vi "Injection.Capture.vi"(7 "FIFOs":T2={"Data Buffer FIFO"="Intermediate Voltage 0", "Capture Complete Trigger FIFO"="Event Capture 0"}, 8 "Current (PreScaled)":fxp<+/-,32,8>, 9 "Voltage (PreScaled)":fxp<+/-,32,8>, 10 "Settings.Index<#>.<Group>.<UserName>":T1, 11 "Settings.Global.<Group>":T3={"Enable?"=FALSE, "Initial Voltage Threshold"=12.0, "Event Dwell Limit"=2000, "Voltage Gain"=1.0, "Current Gain"=1.0, "Filter Samples"=5, "Pretrigger Samples"=5, "Active Edge"=TRUE}) -> (0 "Current (Scaled)":fxp<+/-,32,8>, 1 "Voltage (Scaled)":fxp<+/-,32,8>, 3 "Intermediate FIFO Timeout?":bool)   [LabVIEW 2019]
uses:
  Types/Injection.Global.Settings.ctl
  Types/Injection.Core.Internal.Settings.ctl
  Types/Injection.Core.Settings.ctl
  Types/Injection.Core.State.ctl
  <vilib>/rvi/Emulation/niFpgaSctlEmulationGetInTimedLoop.vi
  <vilib>/Utility/error.llb/Clear Errors.vi
  <vilib>/rvi/DataTransferAndStorage/Container/Common/niFpgaContainerExecOnDevCompGetState.vi
  <vilib>/rvi/Emulation/niFpgaEmulationIsFPGAContextNoSignature.vi
  <vilib>/rvi/errors/niFpgaSetErrorForExecOnDevCompSimple.vi
  <vilib>/rvi/eio/common/nirviEmuReportErrorAndStop.vi
  <vilib>/rvi/DataTransferAndStorage/Container/Common/niFpgaContainerGetUniqueNameForEmu.vi
  <vilib>/rvi/FIFO/Fifo_Resource/nirvififoEmulationSetSize.vi
  <vilib>/rvi/FIFO/Fifo_Resource/nirviFifoEmulationQueueMgr.vi
  <instcachedir>/0/nirviFifoEmulationQueueMgr_E5CAEC123FF24DC58D834DCA3CDAA9B5.lvgen/nirviFifoEmulationQueueMgr_E5CAEC123FF24DC58D834DCA3CDAA9B5_002.vi
  <vilib>/rvi/FIFO/Fifo_Resource/nirvififoEmulationDetermineInputValidOut.vi
  <vilib>/rvi/FIFO/Fifo_Resource/nirvififoEmulationCreateLock.vi
  <vilib>/rvi/Emulation/niFpgaProcessEmulError.vi
  <vilib>/rvi/FIFO/Fifo_Resource/nirvififoEmulationObtainLock.vi
  <vilib>/rvi/FIFO/Fifo_Resource/nirvififoEmulationReleaseLock.vi
  <vilib>/rvi/occurrence/nirviWaitOnOccurrenceBase.vi
  <vilib>/rvi/errors/nirviReportUnexpectedCaseInternalError.vi
  <vilib>/rvi/errors/nirviReportUnexpectedCaseInternalError (U32).vi
  <vilib>/rvi/interface/RandomDataEmulation/niFpgaRandomDataHandleErrors.vi
  <instcachedir>/0/nirviFifoEmulationQueueMgr_E5CAEC123FF24DC58D834DCA3CDAA9B5.lvgen/nirviFifoEmulationQueueMgr_E5CAEC123FF24DC58D834DCA3CDAA9B5_001.vi
  <vilib>/rvi/FXPMathLib/FxpMul/XNode/nifxpmath_Multiplier.xnode
  <vilib>/rvi/FXPMathLib/FxpAdd/XNode/nifxpmath_Add.xnode
  <vilib>/rvi/DataTransferAndStorage/Container/XNode/niFpgaContainer.xnode
  <vilib>/rvi/FIFO/Fifo_Resource/niFpgaFifoEmulationRefIn.vi
  <vilib>/rvi/FXPMathLib/sim/FxpSim.dll
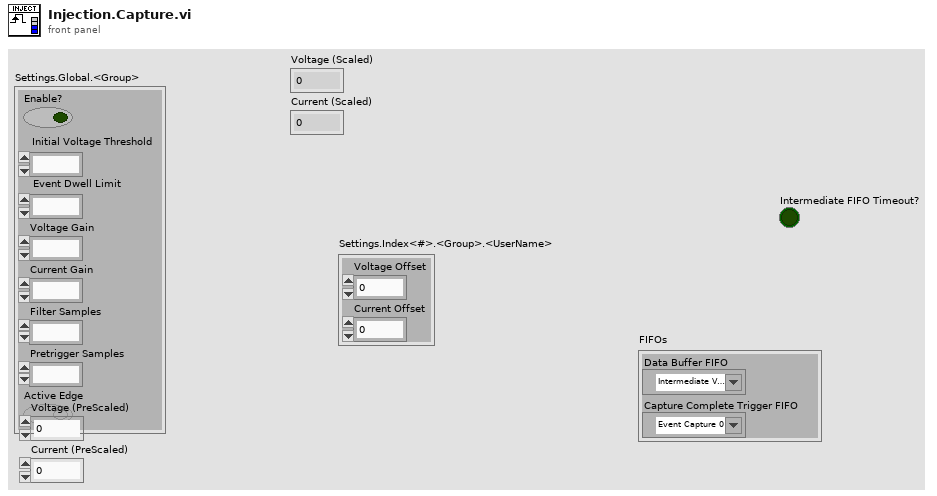
[diagram p1: front panel]
types:
  T1 = typedef "Injection.Core.Settings.ctl" = cluster{"Voltage Offset":fxp<+/-,32,8>, "Current Offset":fxp<+/-,32,8>}
  T2 = typedef "Injection.Core.Internal.Settings.ctl" = cluster{"Data Buffer FIFO":refnum<k21>, "Capture Complete Trigger FIFO":refnum<k21>}
  T3 = typedef "Injection.Global.Settings.ctl" = cluster{"Enable?":bool, "Initial Voltage Threshold":fxp<+/-,32,8>, "Event Dwell Limit":u16, "Voltage Gain":fxp<+/-,32,8>, "Current Gain":fxp<+/-,32,8>, "Filter Samples":u8, "Pretrigger Samples":u8, "Active Edge":bool}
  T4 = cluster{"Event.Count":u16, "Injection.Period":u32, "Injection.CachedPeriod":u32}
  T5 = typedef "Injection.Core.State.ctl" = enum8{"Wait for Start", "Capture Event"}
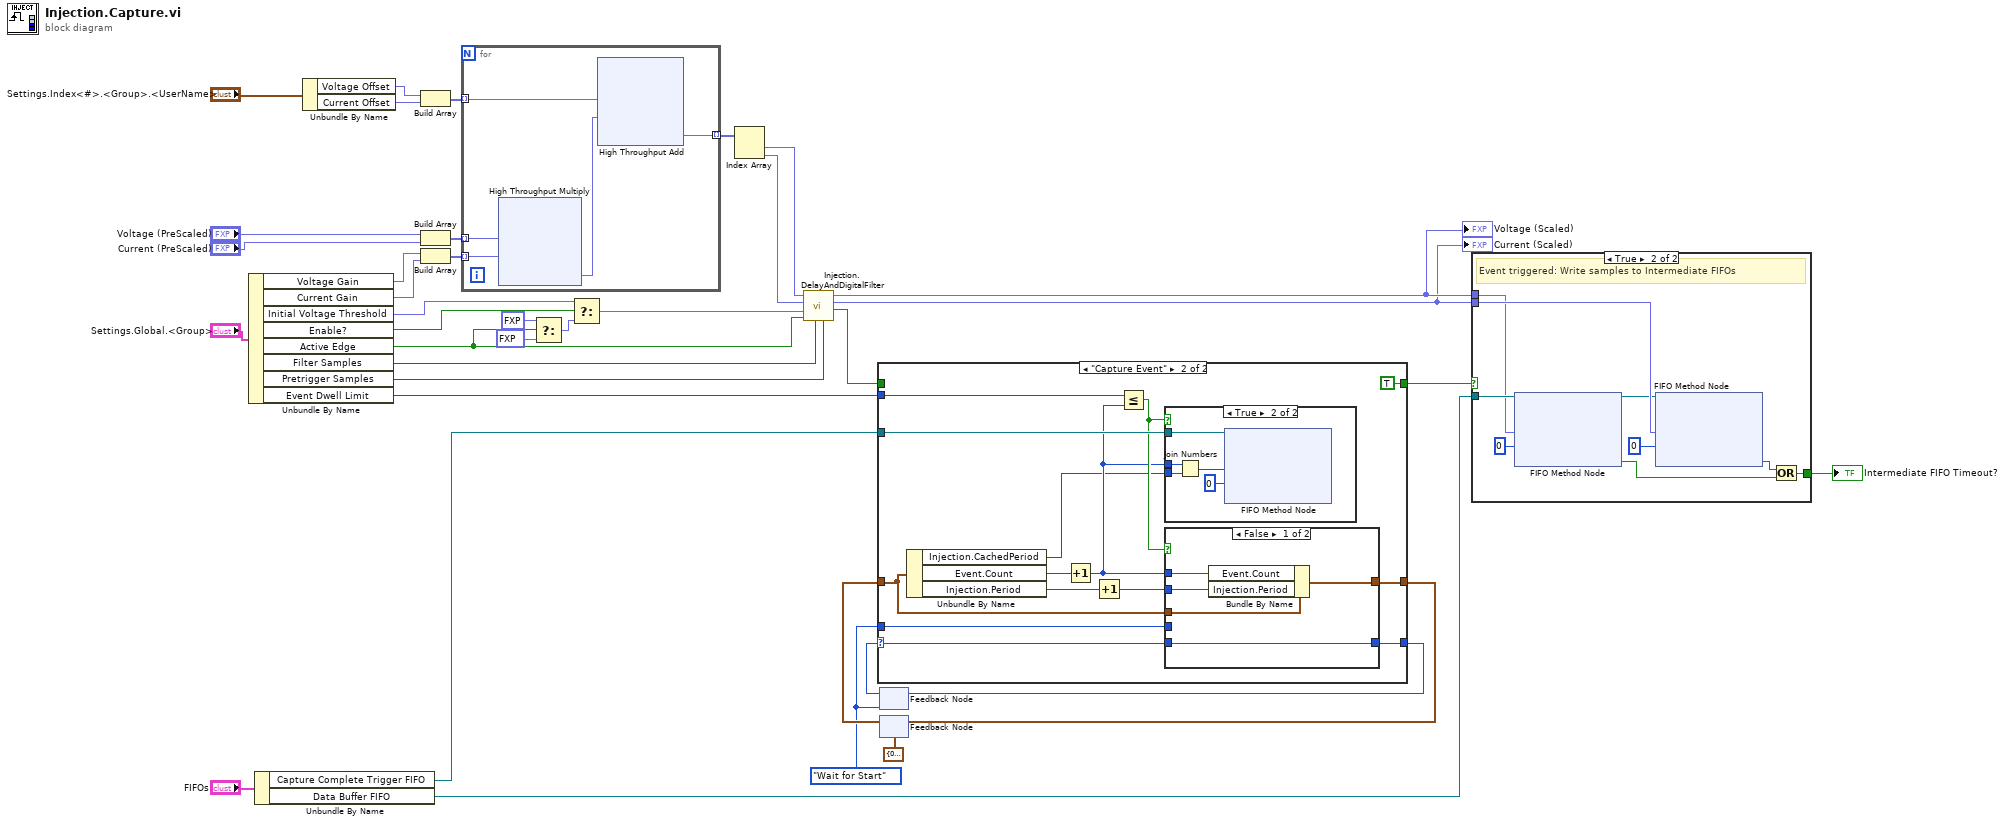
[diagram p0: block diagram]
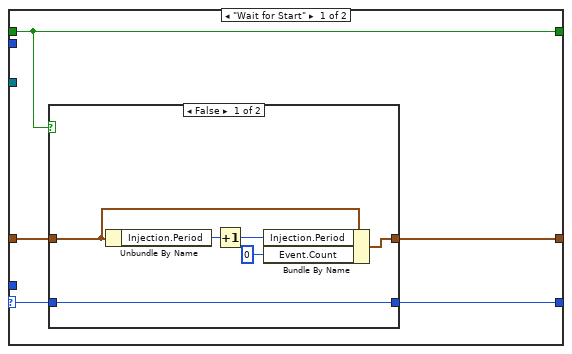
[diagram p2: hidden frame]
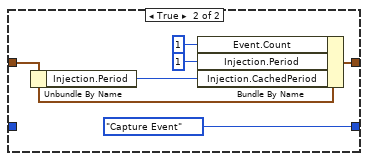
[diagram p3: hidden frame]
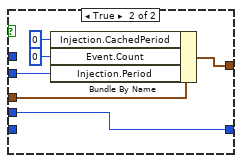
[diagram p5: hidden frame]
diagram:
  w25 = Injection.Core.State."Wait for Start"
  n1 = Unbundle By Name("Settings.Global.<Group>") -> ("Voltage Gain"=w9:fxp<+/-,32,8>, "Current Gain"=w8:fxp<+/-,32,8>, "Initial Voltage Threshold"=w33:fxp<+/-,32,8>, "Enable?"=w34:bool, "Active Edge"=w4:bool, "Filter Samples"=w7:u8, "Pretrigger Samples"=w6:u8, "Event Dwell Limit"=w28:u16)
  n2 = Unbundle By Name("FIFOs") -> ("Capture Complete Trigger FIFO"=w10:refnum<k21>, "Data Buffer FIFO"=w35:refnum<k21>)
  n3 = Unbundle By Name("Settings.Index<#>.<Group>.<UserName>") -> ("Voltage Offset"=w23:fxp<+/-,32,8>, "Current Offset"=w24:fxp<+/-,32,8>)
  n4 = Build Array(w23, w24) -> (w22:fxp<+/-,32,8>[])
  n5 = Build Array("Voltage (PreScaled)", "Current (PreScaled)") -> (w20:fxp<+/-,32,8>[])
  n6 = Build Array(w9, w8) -> (w21:fxp<+/-,32,8>[])
  n7 = for {
    tunnel: w20 -> [w43] mode=indexing
    tunnel: [w39] -> w19 mode=indexing
    tunnel: w22 -> [w41] mode=indexing
    tunnel: w21 -> [w42] mode=indexing
    n8 = xnode ("High Throughput Multiply")("x"=w43, "y"=w42) -> ("x*y"=w40:fxp<+/-,32,8>)
    n9 = xnode ("High Throughput Add")("x"=w41, "y"=w40) -> ("x+y"=w39:fxp<+/-,32,8>)
  }
  n10 = Select(t=fxp<+/-,32,8> 127.99999994039536 ("f"), s=w4, f=fxp<+/-,32,8> -128.0) -> (s? t:f=w1:fxp<+/-,32,8>)
  n11 = Select(t=w33, s=w34, f=w1) -> (s? t:f=w5:fxp<+/-,32,8>)
  n12 = Index Array(array=w19) -> (element #1=w14:fxp<+/-,32,8>, element #2=w13:fxp<+/-,32,8>)  [unwired: 2 in]
  n13 = call "Injection.DelayAndDigitalFilter.vi"("Pretrigger Samples"=w6, "Cycles to Filter"=w7, "Active Edge"=w4, "Threshold"=w5, "Current (PreScaled)"=w13, "Voltage (PreScaled)"=w14) -> ("Output Filtered Signal"=w15:bool, "Current (PreScaled)"=w11:fxp<+/-,32,8>, "Voltage (PreScaled)"=w12:fxp<+/-,32,8>)  [unwired: 3 in]
  "Current (Scaled)" <- w11
  "Voltage (Scaled)" <- w12
  n14 = feedback #1(w25) -> (w32:T5)
  n15 = feedback #2(T4 {"Event.Count"=0, "Injection.Period"=0, "Injection.CachedPeriod"=0}) -> (w30:T4)
  n16 = case shown="\"Capture Event\"" w32 {
    selector: w32 -> [w47 w67]
    tunnel: w15 -> [w45 _]
    tunnel: w30 -> [w48 w72]
    tunnel: [w46 w69] -> w29
    tunnel: w28 -> [_ w64]
    tunnel: [w45 TRUE] -> w27
    tunnel: [w44 w70] -> w26
    tunnel: w25 -> [_ w68]
    tunnel: w10 -> [_ w66]
    frame "Wait for Start" {
      n17 = case shown="False" w45 {
        tunnel: w48 -> [w53 w60]
        tunnel: w47 -> [w54 _]
        tunnel: [w54 Injection.Core.State."Capture Event"] -> w46
        tunnel: [w52 w58] -> w44
        frame False {
          n18 = Unbundle By Name(w53) -> ("Injection.Period"=w50:u32)
          n19 = Increment(x=w50) -> (x+1=w51:u32)
          n20 = Bundle By Name(cluster=w53, "Injection.Period"=w51, "Event.Count"=u32 0) -> (w52:T4)
        }
        frame True {
          n21 = Unbundle By Name(w60) -> ("Injection.Period"=w56:u32)
          n22 = Bundle By Name(cluster=w60, "Event.Count"=u16 1, "Injection.Period"=u32 1 ("Event.Count"), "Injection.CachedPeriod"=w56) -> (w58:T4)
        }
      }
    }
    frame "Capture Event" {
      n23 = Unbundle By Name(w72) -> ("Injection.CachedPeriod"=w61:u32, "Event.Count"=w74:u16, "Injection.Period"=w73:u32)
      n24 = Increment(x=w74) -> (x+1=w62:u16)
      n25 = Increment(x=w73) -> (x+1=w71:u32)
      n26 = Less Or Equal?(x=w64, y=w62) -> (x <= y?=w65:bool)
      n27 = case shown="True" w65 {
        tunnel: w62 -> [_ w76]
        tunnel: w66 -> [_ w79]
        tunnel: w61 -> [_ w77]
        frame False {
        }
        frame True {
          n28 = Join Numbers(hi=w76, lo=w77) -> ((hi.lo)=w75:u64)
          n29 = xnode ("FIFO Method Node")("Element"=w75, "Timeout"=0, "FIFO In"=w79) -> ()  [unwired: 2 out]
        }
      }
      n30 = case shown="False" w65 {
        tunnel: w72 -> [w84 w90]
        tunnel: w71 -> [w83 w88]
        tunnel: [w82 w89] -> w70
        tunnel: w62 -> [w81 _]
        tunnel: [w80 w86] -> w69
        tunnel: w68 -> [_ w86]
        tunnel: w67 -> [w80 _]
        frame False {
          n31 = Bundle By Name(cluster=w84, "Event.Count"=w81, "Injection.Period"=w83) -> (w82:T4)
        }
        frame True {
          n32 = Bundle By Name(cluster=w90, "Injection.CachedPeriod"=u32 0, "Event.Count"=u16 0, "Injection.Period"=w88) -> (w89:T4)
        }
      }
    }
  }
  n33 = feedback-in #1(w29) -> ()
  n34 = feedback-in #2(w26) -> ()
  n35 = case shown="True" w27 {
    tunnel: w12 -> [_ w92]
    tunnel: [_ w94] -> w37
    tunnel: w11 -> [_ w97]
    tunnel: w35 -> [_ w98]
    frame False {
      # "Event is not triggered"
    }
    frame True {
      # "Event triggered: Write samples to Intermediate FIFOs"
      n36 = xnode ("FIFO Method Node")("Element"=w92, "Timeout"=0 ("timeout in ms (0)"), "FIFO In"=w98) -> ("Timed Out?"=w95:bool, "FIFO Out"=w91:refnum<k21>)  [unwired: 1 in, 1 out]
      n37 = xnode ("FIFO Method Node")("Element"=w97, "Timeout"=0 ("timeout in ms (0)"), "FIFO In"=w91) -> ("Timed Out?"=w93:bool)  [unwired: 1 in, 2 out]
      n38 = Or(x=w93, y=w95) -> (x .or. y?=w94:bool)
    }
  }
  "Intermediate FIFO Timeout?" <- w37
